vi "Write ModuleName.vi"(8 "error in (no error)":errorcluster, 10 "ModuleName":string, 11 "DAQ_Module in":refnum<class "DAQ_Module.lvclass">) -> (0 "error out":errorcluster, 3 "DAQ_Module out":refnum<class "DAQ_Module.lvclass">)   [LabVIEW 2025, in "DAQ_Module.lvlib" / "DAQ_Module.lvclass"]
uses:
  DAQ_Module.lvclass
  DAQ_Module.lvclass/DAQ_Module.ctl
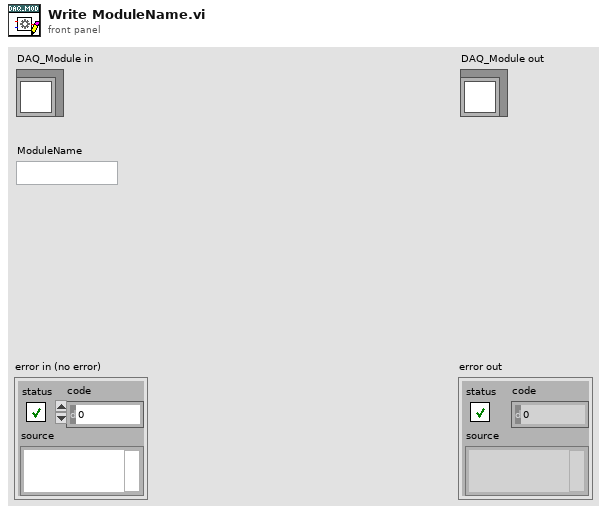
[diagram p1: front panel]
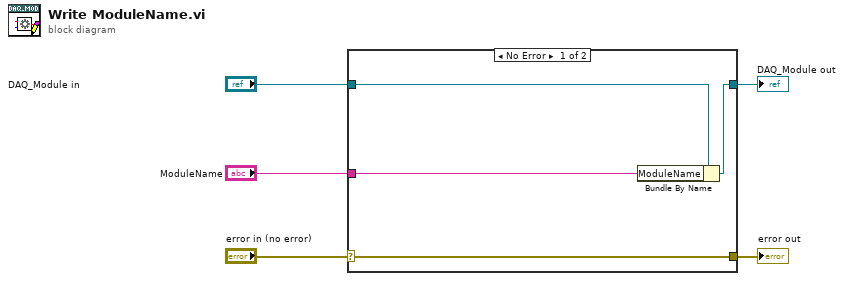
[diagram p0: block diagram]
diagram:
  n1 = case shown="No Error" "error in (no error)" {
    selector: "error in (no error)" -> [w9 w10]
    tunnel: [w9 w10] -> w4
    tunnel: [w7 w11] -> w2
    tunnel: "DAQ_Module in" -> [w8 w11]
    tunnel: "ModuleName" -> [w6 _]
    frame No Error {
      n2 = Bundle By Name(cluster=w8, "ModuleName"=w6) -> (w7:refnum<class "DAQ_Module.lvclass">)
    }
    frame Error {
    }
  }
  "error out" <- w4
  "DAQ_Module out" <- w2
